vi "Check Data Model.vi"(8 "error in (no error)":errorcluster, 11 "device data model in":refnum<class "WebSocket Data Model.lvclass">) -> (0 "error out":errorcluster, 3 "device data model out":refnum<class "WebSocket Data Model.lvclass">)   [LabVIEW 2021, in "WebSockets.lvlib" / "WebSocket Data Model.lvclass"]
doc: "This VI ensures that the data model has at least 65,535 values of every type. This is required for certain modbus function codes."
uses:
  WebSocket Data Model.lvclass
  WebSocket Data Model.lvclass/WebSocket Data Model.ctl
  Type Definitions/Data Model.ctl
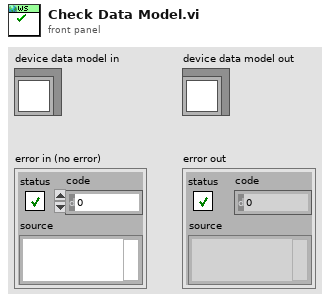
[diagram p1: front panel]
types:
  T1 = typedef "WebSockets.lvlib/WebSocket Data Model.lvclass/Data Model.ctl" = cluster{"UTC":u64, "Receive Binary Data":u8[], "Receive Text Data":string, "Send Binary Data":u8[], "Send Text Data":string, "ES":u8}
  T2 = typedef "Device Data Model.lvclass/N channel.ctl" = cluster{"N DI channel":i32, "N DO channel":i32, "N AI channel":i32, "N AO channel":i32}
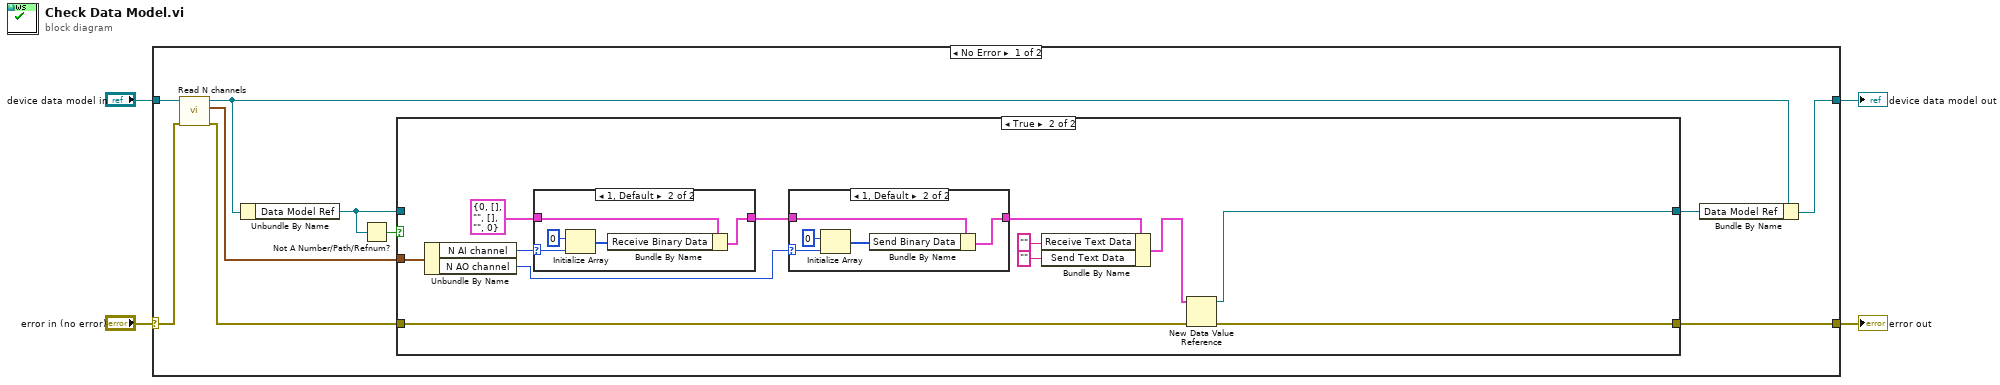
[diagram p0: block diagram]
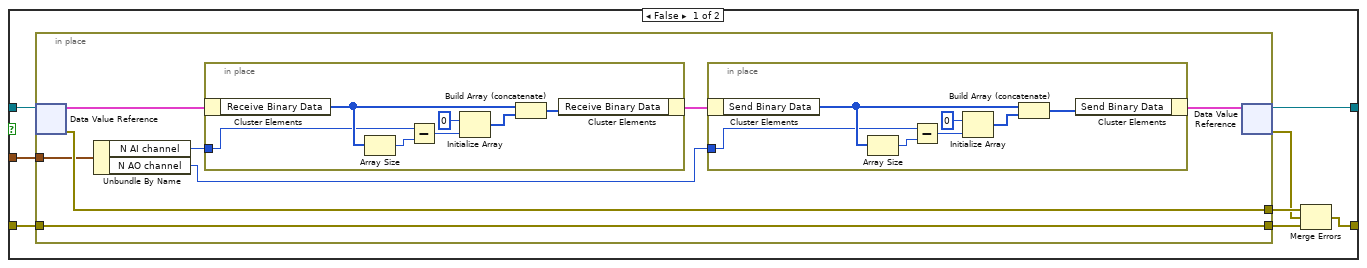
[diagram p2: hidden frame]
diagram:
  n1 = case shown="No Error" "error in (no error)" {
    selector: "error in (no error)" -> [w7 w70]
    tunnel: "device data model in" -> [w9 w69]
    tunnel: [w14 w69] -> w3
    tunnel: [w10 w70] -> w2
    frame No Error {
      n2 = call-dynamic "Read N channels.vi"("error in (no error)"=w7, "device data model in"=w9) -> ("error out"=w6:errorcluster, "N channel"=w5:T2, "device data model out"=w8:refnum<class "WebSocket Data Model.lvclass">)  [unwired: 7 in]
      n3 = Unbundle By Name(w8) -> ("Data Model Ref"=w12:refnum<data-value>)
      n4 = Not A Number/Path/Refnum?(number/path/refnum=w12) -> (NaN/Path/Refnum?=w11:bool)
      n5 = case shown="True" w11 {
        tunnel: w6 -> [w22 w56]
        tunnel: w12 -> [w21 _]
        tunnel: [w20 w54] -> w13
        tunnel: [w18 w55] -> w10
        tunnel: w5 -> [w15 w51]
        frame False {
          n6 = in-place {
            in-place-border: w22 -> [w28]
            in-place-border: [w29] -> w19
            in-place-border: [w28] -> w16
            in-place-border: w15 -> [w27]
            n7 = in-place-dvr #1(w21) -> (w30:T1, w29:errorcluster)
            n8 = Unbundle By Name(w27) -> ("N AI channel"=w26:i32, "N AO channel"=w24:i32)
            n9 = in-place {
              in-place-border: w26 -> [w38]
              n10 = in-place-cluster #2(w30) -> ("Receive Binary Data"=w41:u8[])
              n11 = Array Size(array=w41) -> (size(s)=w44:i32)
              n12 = Subtract(x=w38, y=w44) -> (x-y=w43:i32)
              n13 = Initialize Array(u8 0 ("Boolean"), w43) -> (w42:u8[])
              n14 = Build Array (concatenate)(w41, w42) -> (w39:u8[])
              n15 = in-place-cluster #2("Receive Binary Data"=w39) -> (w25:T1)
            }
            n16 = in-place {
              in-place-border: w24 -> [w31]
              n17 = in-place-cluster #3(w25) -> ("Send Binary Data"=w34:u8[])
              n18 = Array Size(array=w34) -> (size(s)=w37:i32)
              n19 = Subtract(x=w31, y=w37) -> (x-y=w36:i32)
              n20 = Initialize Array(u8 0 ("Boolean"), w36) -> (w35:u8[])
              n21 = Build Array (concatenate)(w34, w35) -> (w32:u8[])
              n22 = in-place-cluster #3("Send Binary Data"=w32) -> (w23:T1)
            }
            n23 = in-place-dvr #1(w23) -> (w20:refnum<data-value>, w17:errorcluster)
          }
          n24 = Merge Errors(w19, w17, w16) -> (w18:errorcluster)
        }
        frame True {
          n25 = Unbundle By Name(w51) -> ("N AI channel"=w52:i32, "N AO channel"=w45:i32)
          n26 = case shown="1, Default" w52 {
            selector: w52 -> [_ w64]
            tunnel: T1 {"UTC"=0, "Receive Binary Data"=[], "Receive Text Data"="", "Send Binary Data"=[], "Send Text Data"="", "ES"=0} ("Data Model") -> [w63 w67]
            tunnel: [w63 w65] -> w47
            frame 0 {
            }
            frame 1, Default {
              n27 = Initialize Array(u8 0 ("Boolean"), w64) -> (w66:u8[])
              n28 = Bundle By Name(cluster=w67, "Receive Binary Data"=w66) -> (w65:T1)
            }
          }
          n29 = case shown="1, Default" w45 {
            selector: w45 -> [_ w58]
            tunnel: w47 -> [w57 w61]
            tunnel: [w57 w59] -> w46
            frame 0 {
            }
            frame 1, Default {
              n30 = Initialize Array(u8 0 ("Boolean"), w58) -> (w60:u8[])
              n31 = Bundle By Name(cluster=w61, "Send Binary Data"=w60) -> (w59:T1)
            }
          }
          n32 = Bundle By Name(cluster=w46, "Receive Text Data"="" ("Text Data"), "Send Text Data"="" ("Text Data")) -> (w50:T1)
          n33 = New Data Value Reference(data value=w50, error in=w56) -> (data value reference=w54:refnum<data-value>, error out=w55:errorcluster)
        }
      }
      n34 = Bundle By Name(cluster=w8, "Data Model Ref"=w13) -> (w14:refnum<class "WebSocket Data Model.lvclass">)
    }
    frame Error {
    }
  }
  "error out" <- w2
  "device data model out" <- w3
